vi "PollDataBindBoolbyNm.vi"(6 "Timeout(ms)":i32=-1, 7 "Valeur":bool=TRUE, 8 "error in":errorcluster caption="entrée d'erreur", 9 "TargetName":string="LaserLowTime", 10 "DataBindCtrlNm":string[](array[string]), 11 "Control Ref":refnum<vi>[](array[refnum])) -> (0 "error out":errorcluster caption="sortie d'erreur", 3 "Timeout":bool)   [LabVIEW 2019]
uses:
  <userlib>/GenProg/T_At_Wire/T_At_Wire_Err.vi
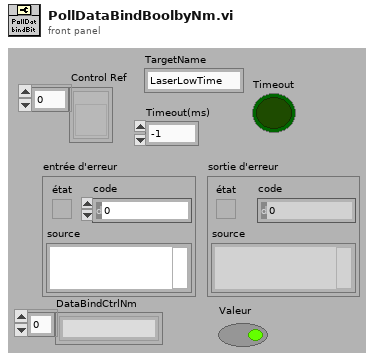
[diagram p1: front panel]
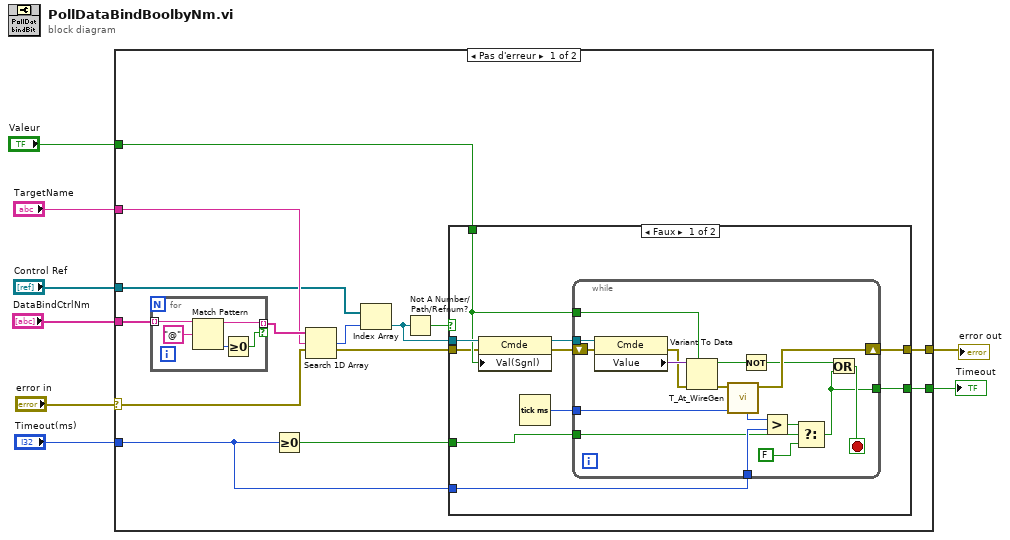
[diagram p0: block diagram]
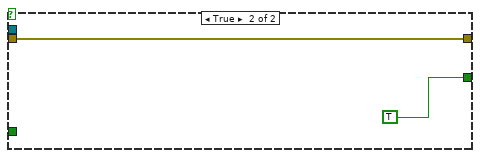
[diagram p2: hidden frame]
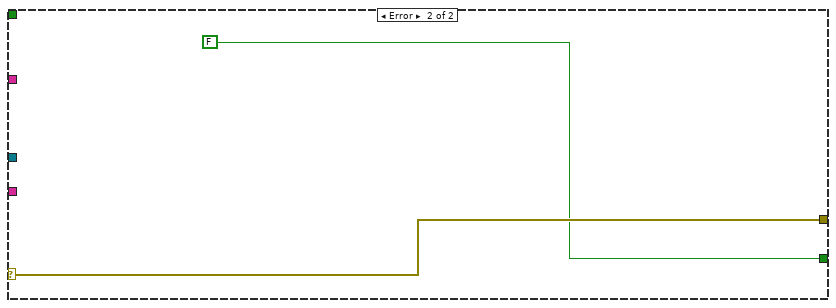
[diagram p3: hidden frame]
diagram:
  n1 = case shown="Pas d'erreur" "error in" {
    selector: "error in" -> [w15 w57]
    tunnel: "Control Ref" -> [w12 _]
    tunnel: [w11 FALSE ("Value")] -> w7
    tunnel: [w14 w57] -> w5
    tunnel: "DataBindCtrlNm" -> [w17 _]
    tunnel: "TargetName" -> [w16 _]
    tunnel: "Valeur" -> [w13 _]
    tunnel: "Timeout(ms)" -> [w10 _]
    frame No Error {
      n2 = for {
        tunnel: w17 -> [w26] mode=indexing
        tunnel: [w24] -> w18 mode=indexing if=w23
        n3 = Match Pattern(string=w26, regular expression="@" ("expression régulière")) -> (before substring=w24:string, offset past match=w22:i32)  [unwired: 1 in, 2 out]
        n4 = Greater Or Equal To 0?(x=w22) -> (x >= 0?=w23:bool)
      }
      n5 = Greater Or Equal To 0?(x=w10) -> (x >= 0?=w9:bool)
      n6 = Search 1D Array(1D array=w18, element=w16) -> (index of element=w21:i32)  [unwired: 1 in]
      n7 = Index Array(array=w12, index=w21) -> (element=w19:refnum<vi>)
      n8 = Not A Number/Path/Refnum?(number/path/refnum=w19) -> (NaN/Path/Refnum?=w20:bool)
      n9 = case shown="Faux" w20 {
        tunnel: w19 -> [w36 _]
        tunnel: w15 -> [w28 w55]
        tunnel: [w30 w55] -> w14
        tunnel: w13 -> [w33 _]
        tunnel: w10 -> [w31 _]
        tunnel: [w29 TRUE] -> w11
        tunnel: w9 -> [w27 _]
        frame False {
          n10 = property class="Cmde"(reference=w36, error in=w28, "Val(Sgnl)"=w33) -> (reference out=w35:refnum<vi>, error out=w34:errorcluster)
          n11 = Tick Count (ms)() -> (millisecond timer value=w32:u32)
          n12 = while {
            tunnel: w35 -> [w53]
            tunnel: w33 -> [w50]
            shift-right: [w46] -> w30
            shift-left: w34 -> [w52]
            tunnel: w32 -> [w45]
            tunnel: w31 -> [w43]
            tunnel: [w40] -> w29
            tunnel: w27 -> [w39]
            stop <- w41 stop-if-true
            n13 = property class="Cmde"(reference=w53, error in=w52) -> (error out=w48:errorcluster, "Value"=w51:variant)  [unwired: 1 out]
            n14 = Variant To Data(error in=w48, type=w50, Variant=w51) -> (data=w47:bool, error out=w49:errorcluster)
            n15 = call-poly <userlib>:"T_At_WireGen.vi"("InitClock(ms)"=w45, "error in (no error)"=w49) -> ("error out"=w46:errorcluster, "Delta(ms)"=w44:u32)  [unwired: 7 in, 1 out]
            n16 = Not(x=w47) -> (.not. x?=w42:bool)
            n17 = Greater?(x=w44, y=w43) -> (0:w38:bool)
            n18 = Select(t=w38, s=w39, f=FALSE ("cas faux")) -> (s? t:f=w40:bool)
            n19 = Or(x=w42, y=w40) -> (x .or. y?=w41:bool)
          }
        }
        frame True {
        }
      }
    }
    frame Error {
    }
  }
  "Timeout" <- w7
  "error out" <- w5
